vi "HTSuperProWriteDigital.vi"(0 "Digital Value":u8, 3 "NXT":T1, 4 "Port":T2 items=["Port 1", "Port 2", "Port 3", "Port 4"]) -> (5 "NXT":T1)   [LabVIEW 2012]
doc: "HiTechnic SuperPro - Write Digital Port\n\n<B>Inputs\nPort </B> is the port connected to the sensor. Port 1 is the default, but Port 2, Port 3, or Port 4 can also be selected.\n<B>NXT </B> connects to NXT terminal of previous VI to establish the flow of the program.\n<B>Digital Value</B> value to be written to the digital B7-B0 pins on the SuperPro. Note that you must configure bits for output using HTSuperProWriteControl .\n\n<B>Outputs\nNXT </B> wires to NXT terminal of next VI to establish the flow of the program."
uses:
  <vilib>/NXT/Block Support/NXT_InputPort.ctl
  <vilib>/NXT/Subs/LVHSConnector.ctl
  <vilib>/NXT/LegoClasses/BrickReference/BrickReference.lvclass
  <vilib>/NXT/Block Support/HWPage.SensorType.ctl
  <vilib>/NXT/Block Support/HWPage.SensorMode.ctl
panel:
  # "HiTechnic SuperPro Prototype board VI\nWrite Digital Port\n\nWrite to the digital B0 to B7 pins.  Note that only bits set to 1 in the control byte will actually be available for output. \n\n(c) HiTechnic 2011"
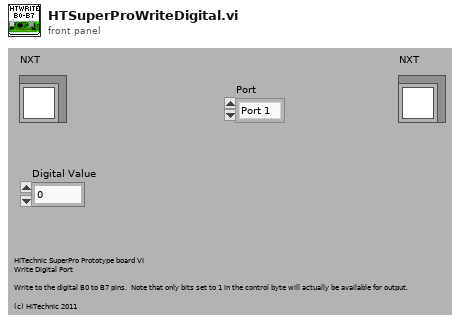
[diagram p1: front panel]
types:
  T1 = typedef "LVHSConnector.ctl" = refnum<class "BrickReference.lvclass">
  T2 = typedef "NXT_InputPort.ctl" = u32
  T3 = typedef "HWPage.SensorType.ctl" = u8
  T4 = typedef "HWPage.SensorMode.ctl" = u8
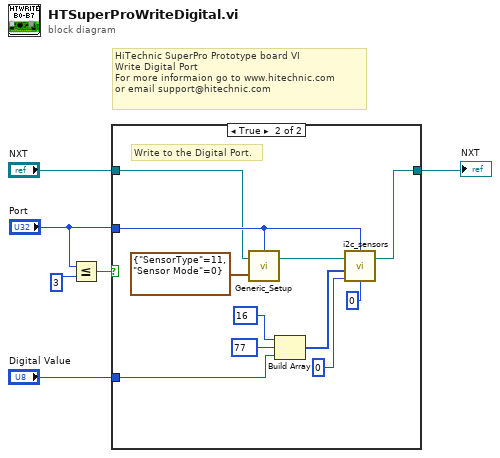
[diagram p0: block diagram]
diagram:
  # "HiTechnic SuperPro Prototype board VI\nWrite Digital Port\nFor more informaion go to www.hitechnic.com\nor email support@hitechnic.com"
  n1 = Less Or Equal?(x="Port", y=u8 3) -> (x <= y?=w2:bool)
  n2 = case shown="True" w2 {
    tunnel: "Port" -> [_ w17]
    tunnel: "NXT" -> [w7 w16]
    tunnel: [w7 w14] -> w4
    tunnel: "Digital Value" -> [_ w9]
    frame False {
    }
    frame True {
      # "Write to the Digital Port."
      n3 = call <vilib>:"Generic_Setup.vi"("Sensor Setup"=cluster{"SensorType":T3, "Sensor Mode":T4} {"SensorType"=11, "Sensor Mode"=0}, "NXT/EV3"=w16, "Port"=w17) -> ("NXT/EV3"=w15:T1)  [unwired: 1 out]
      n4 = Build Array(u8 16, u8 77, w9) -> (w12:u8[])
      n5 = call <vilib>:"i2c_sensors.vi"("Return Length"=u8 0, "Bytes to Write"=w12, "Wait (msec)"=u32 0, "NXT/EV3"=w15, "Port"=w17) -> ("NXT/EV3"=w14:T1)  [unwired: 2 out]
    }
  }
  "NXT" <- w4
